vi "Open Camera.vi"(8 "error in (no error)":errorcluster, 10 "Camera ID":i32, 11 "Picam in":refnum<class "Picam.lvclass">) -> (0 "error out":errorcluster, 2 "Camera Detected":bool, 3 "Picam out":refnum<class "Picam.lvclass">)   [LabVIEW 2019, in "Picam.lvclass"]
uses:
  Picam.lvclass
  Picam.lvclass/Picam.ctl
  <vilib>/Utility/error.llb/Error Cluster From Error Code.vi
  <vilib>/ErrorRing/Error Ring.xnode
  picam32_LabView_SDK/PICam_lib/PICam.lvlib
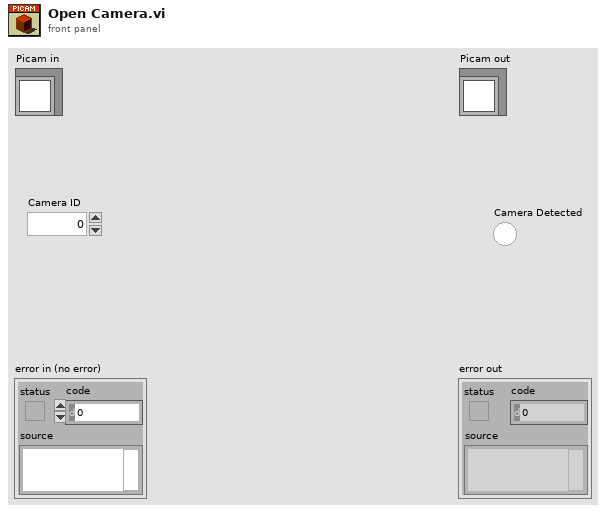
[diagram p1: front panel]
types:
  T1 = typedef "PICam.lvlib/PicamCameraID.ctl" = cluster{"PicamModel":T2, "PicamComputerInterface":T3, "sensor_name":T4, "serial_number":T5}
  T2 = typedef "PICAM.lvlib/PicamModel.ctl" = u32
  T3 = typedef "PICAM.lvlib/PicamComputerInterface.ctl" = u32
  T4 = typedef "PICAM.lvlib/sensor_name.ctl" = cluster{"U8":u8, "U8 2":u8, "U8 3":u8, "U8 4":u8, "U8 5":u8, "U8 6":u8, "U8 7":u8, "U8 8":u8, "U8 9":u8, "U8 10":u8, "U8 11":u8, "U8 12":u8, "U8 13":u8, "U8 14":u8, "U8 15":u8, "U8 16":u8, "U8 17":u8, "U8 18":u8, "U8 19":u8, "U8 20":u8, "U8 21":u8, "U8 22":u8, "U8 23":u8, "U8 24":u8, "U8 25":u8, "U8 26":u8, "U8 27":u8, "U8 28":u8, "U8 29":u8, "U8 30":u8, "U8 31":u8, "U8 32":u8, "U8 33":u8, "U8 34":u8, "U8 35":u8, "U8 36":u8, "U8 37":u8, "U8 38":u8, "U8 39":u8, "U8 40":u8, "U8 41":u8, "U8 42":u8, "U8 43":u8, "U8 44":u8, "U8 45":u8, "U8 46":u8, "U8 47":u8, "U8 48":u8, "U8 49":u8, "U8 50":u8, "U8 51":u8, "U8 52":u8, "U8 53":u8, "U8 54":u8, "U8 55":u8, "U8 56":u8, "U8 57":u8, "U8 58":u8, "U8 59":u8, "U8 60":u8, "U8 61":u8, "U8 62":u8, "U8 63":u8, "U8 64":u8}
  T5 = typedef "PICAM.lvlib/serial_number.ctl" = cluster{"U8":u8, "U8 2":u8, "U8 3":u8, "U8 4":u8, "U8 5":u8, "U8 6":u8, "U8 7":u8, "U8 8":u8, "U8 9":u8, "U8 10":u8, "U8 11":u8, "U8 12":u8, "U8 13":u8, "U8 14":u8, "U8 15":u8, "U8 16":u8, "U8 17":u8, "U8 18":u8, "U8 19":u8, "U8 20":u8, "U8 21":u8, "U8 22":u8, "U8 23":u8, "U8 24":u8, "U8 25":u8, "U8 26":u8, "U8 27":u8, "U8 28":u8, "U8 29":u8, "U8 30":u8, "U8 31":u8, "U8 32":u8, "U8 33":u8, "U8 34":u8, "U8 35":u8, "U8 36":u8, "U8 37":u8, "U8 38":u8, "U8 39":u8, "U8 40":u8, "U8 41":u8, "U8 42":u8, "U8 43":u8, "U8 44":u8, "U8 45":u8, "U8 46":u8, "U8 47":u8, "U8 48":u8, "U8 49":u8, "U8 50":u8, "U8 51":u8, "U8 52":u8, "U8 53":u8, "U8 54":u8, "U8 55":u8, "U8 56":u8, "U8 57":u8, "U8 58":u8, "U8 59":u8, "U8 60":u8, "U8 61":u8, "U8 62":u8, "U8 63":u8, "U8 64":u8}
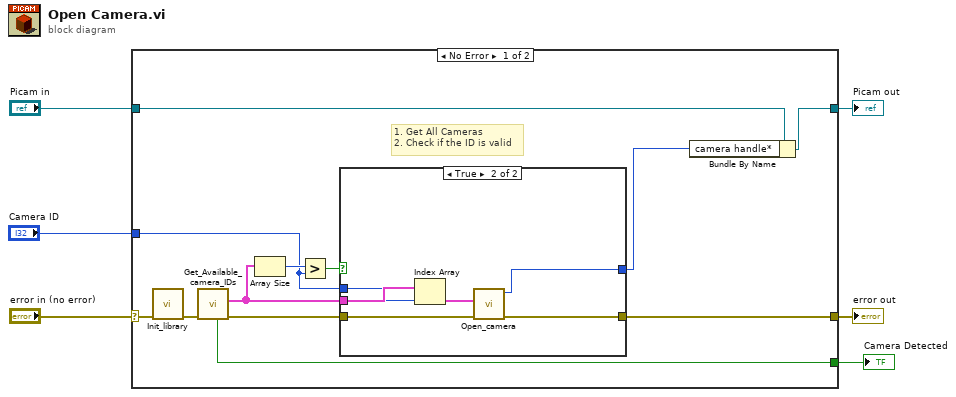
[diagram p0: block diagram]
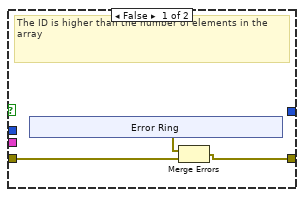
[diagram p2: hidden frame]
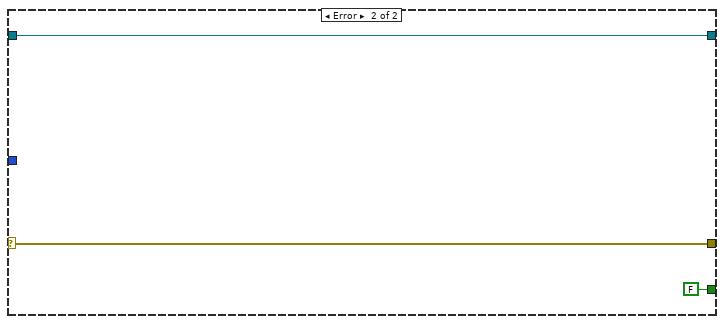
[diagram p3: hidden frame]
diagram:
  n1 = case shown="No Error" "error in (no error)" {
    selector: "error in (no error)" -> [w18 w35]
    tunnel: [w9 w35] -> w5
    tunnel: [w15 w34] -> w3
    tunnel: "Picam in" -> [w16 w34]
    tunnel: "Camera ID" -> [w10 _]
    tunnel: [w7 FALSE ("Camera detected?")] -> w1
    frame No Error {
      # "1. Get All Cameras\n2. Check if the ID is valid"
      n2 = call "Init_library.vi"("error in"=w18) -> ("error out"=w17:errorcluster)  [unwired: 10 in]
      n3 = call "Get_Available_camera_IDs.vi"("error in"=w17) -> ("error out"=w12:errorcluster, "PicamCameraIDs"=w11:T1[], "Camera detected?"=w7:bool)  [unwired: 8 in]
      n4 = Array Size(array=w11) -> (size(s)=w14:i32)
      n5 = Greater?(x=w14, y=w10) -> (0:w13:bool)
      n6 = case shown="True" w13 {
        tunnel: w12 -> [w21 w30]
        tunnel: w11 -> [_ w32]
        tunnel: w10 -> [_ w31]
        tunnel: [w20 w28] -> w9
        tunnel: [_ w27] -> w8
        frame False {
          # "The ID is higher than the number of elements in the array"
          n7 = xnode "Error Ring"() -> ("error out"=w19:errorcluster)
          n8 = Merge Errors(w19, w21) -> (w20:errorcluster)
        }
        frame True {
          n9 = Index Array(array=w32, index=w31) -> (element=w29:T1)
          n10 = call "Open_camera.vi"("error in"=w30, "PicamCameraID"=w29) -> ("error out"=w28:errorcluster, "camera handler out"=w27:u64)  [unwired: 8 in]
        }
      }
      n11 = Bundle By Name(cluster=w16, "camera handle*"=w8) -> (w15:refnum<class "Picam.lvclass">)
    }
    frame Error {
    }
  }
  "error out" <- w5
  "Picam out" <- w3
  "Camera Detected" <- w1
